vi "DoCmd-SetDataMember.vi"(8 "error in (no error)":errorcluster, 10 "Cmd Data":variant, 11 "DVR Cluster In":T1) -> (0 "error out":errorcluster, 3 "DVR Cluster Out":T1)   [LabVIEW 2024, in "GLF.lvlib" / "Engine.lvclass"]
uses:
  Engine.lvclass
  Engine.lvclass/Engine.ctl
  DataMember--enum.ctl
  CommandData-SetDataMember--cluster.ctl
  VSync--enum.ctl
  Config--cluster.ctl
  Context--cluster.ctl
  Metrics--cluster.ctl
  Command--enum.ctl
  Command--cluster.ctl
  Command--queue.ctl
  DVR--cluster.ctl
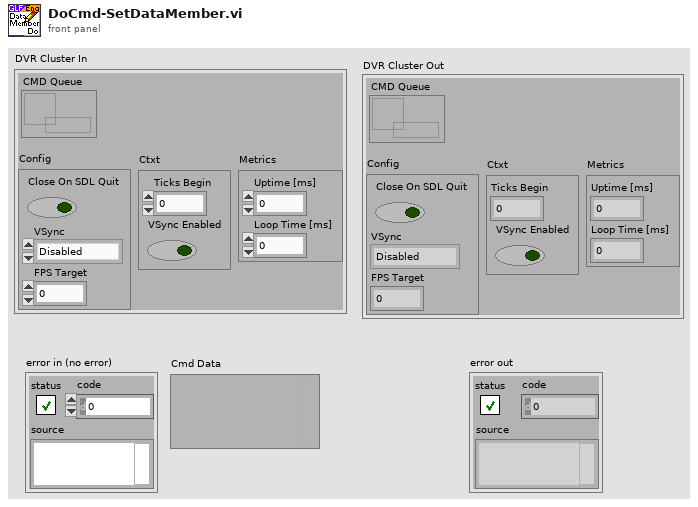
[diagram p1: front panel]
types:
  T1 = typedef "GLF.lvlib/Engine.lvclass/DVR--cluster.ctl" = cluster{"CMD Queue":T2, "Config":T3, "Ctxt":T5, "Metrics":T6}
  T2 = typedef "GLF.lvlib/Engine.lvclass/Command--queue.ctl" = refnum<queue>
  T3 = typedef "GLF.lvlib/Engine.lvclass/Config--cluster.ctl" = cluster{"Close On SDL Quit":bool, "VSync":T4, "FPS Target":dbl}
  T4 = typedef "GLF.lvlib/Engine.lvclass/VSync--enum.ctl" = enum16{"Disabled", "Enabled", "Adaptative"}
  T5 = typedef "GLF.lvlib/Engine.lvclass/Context--cluster.ctl" = cluster{"Ticks Begin":u64, "VSync Enabled":bool}
  T6 = typedef "GLF.lvlib/Engine.lvclass/Metrics--cluster.ctl" = cluster{"Uptime [ms]":u64, "Loop Time [ms]":u64}
  T7 = typedef "GLF.lvlib/Engine.lvclass/CommandData-SetDataMember--cluster.ctl" = cluster{"Data Member":T8, "Value":variant}
  T8 = typedef "GLF.lvlib/Engine.lvclass/DataMember--enum.ctl" = enum16{"Close On SDL Quit?"}
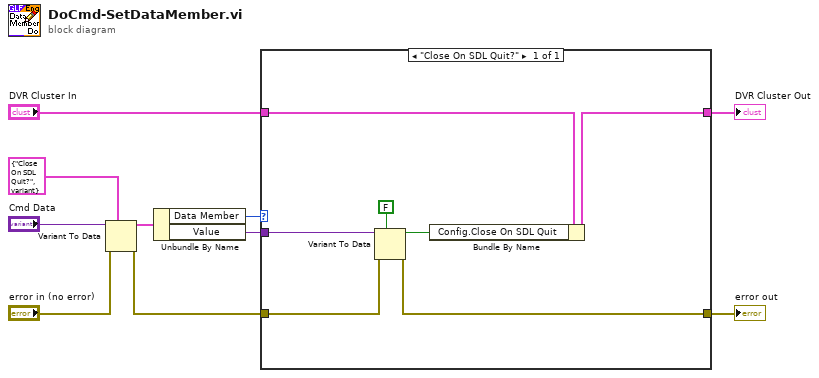
[diagram p0: block diagram]
diagram:
  n1 = Variant To Data(error in="error in (no error)", type=T7 {"Data Member"=enum."Close On SDL Quit?", "Value"=variant} ("Set Data Member Cmd Data"), Variant="Cmd Data") -> (data=w7:T7, error out=w4:errorcluster)
  n2 = Unbundle By Name(w7) -> ("Data Member"=w6:T8, "Value"=w5:variant)
  n3 = case shown="\"Close On SDL Quit?\"" w6 {
    tunnel: "DVR Cluster In" -> [w17]
    tunnel: [w12] -> w1
    tunnel: w5 -> [w16]
    tunnel: w4 -> [w14]
    tunnel: [w15] -> w3
    frame "Close On SDL Quit?" {
      n4 = Variant To Data(error in=w14, type=FALSE, Variant=w16) -> (data=w11:bool, error out=w15:errorcluster)
      n5 = Bundle By Name(cluster=w17, "Config.Close On SDL Quit"=w11) -> (w12:T1)
    }
  }
  "error out" <- w3
  "DVR Cluster Out" <- w1
